vi "Copy Array to Image (Greyscale).vi"(8 "error in (no error)":errorcluster, 10 "Greyscale Destination Image":T1, 11 "U8 Greyscale Data":u8[][](array[numeric])) -> (0 "error out":errorcluster, 3 "Greyscale Destination Image (duplicate)":T1)   [LabVIEW 2020, in "g_ar_toolkit.image.lvlib"]
uses:
  g_ar_toolkit.image.lvlib
  Greyscale Image.ctl
  g_ar_toolkit.common/g_ar_toolkit.common.lvlib
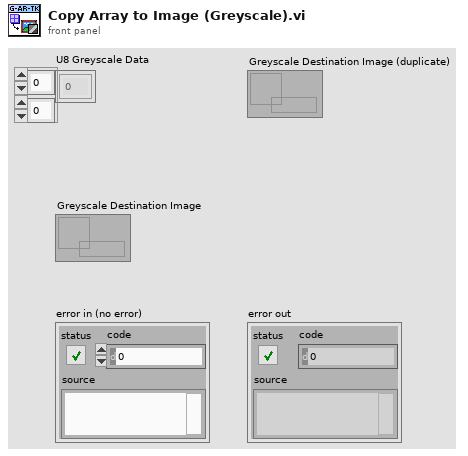
[diagram p1: front panel]
types:
  T1 = typedef "g_ar_toolkit.image.lvlib/Greyscale Image.ctl" = refnum<data-value>
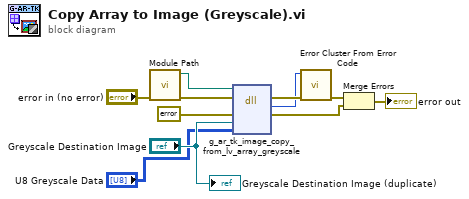
[diagram p0: block diagram]
diagram:
  n1 = call "Module Path.vi"("error in (no error)"="error in (no error)") -> ("error out"=w2:errorcluster, "Path"=w1:path)  [unwired: 9 in]
  n2 = dll-call lib="?" fn="g_ar_tk_image_copy_from_lv_array_greyscale" ("g_ar_toolkit.*.*:g_ar_tk_image_copy_from_raw_memory")(path in=w1, error in=w2, "error_cluster"=errorcluster {"status"=FALSE, "code"=0, "source"=""} ("error constant"), "EDVR Dst"="Greyscale Destination Image", "array"="U8 Greyscale Data") -> (error out=w4:errorcluster, "MgErr"=w3:i32, "error_cluster"=w10:errorcluster)  [unwired: 3 in, 1 out]
  n3 = call <vilib>:"Error Cluster From Error Code.vi"("error in (no error)"=w4, "error code (0)"=w3) -> ("error out"=w5:errorcluster)  [unwired: 7 in]
  n4 = Merge Errors(w5, w10) -> (→"error out":errorcluster)
  "Greyscale Destination Image (duplicate)" <- "Greyscale Destination Image"
